vi "Gergberg Setup.vi"() -> ()   [LabVIEW 2012, in "LightPipes.lvlib"]
uses:
  LightPipes.lvlib
panel:
  in  "Target Phase":path=path "C:/Users/Tri/Documents/Lightpipes/LabView/beam images/target_phase.gpl"
  in  "Target PGM":path=path "C:/Users/Tri/Documents/Lightpipes/LabView/beam images/target.pgm"
  in  "R":dbl=0.0001
  in  "size_grid":dbl=0.02
  in  "n_grid":i32=256
  in  "Source Intensity":path=path "C:/Users/Tri/Documents/Lightpipes/LabView/beam images/initial_int.gpl"
  in  "Target Intensity":path=path "C:/Users/Tri/Documents/Lightpipes/LabView/beam images/target_int.gpl"
  in  "PGM gamma":dbl=1.0
  in  "Source PGM":path=path "C:/Users/Tri/Documents/Lightpipes/LabView/beam images/initial.pgm"
  in  "forward distance":dbl=0.5
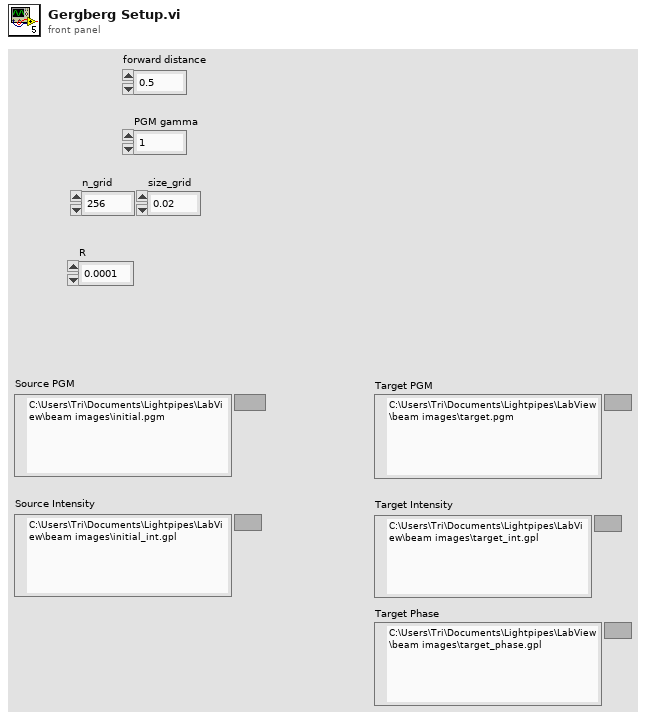
[diagram p1: front panel]
types:
  T1 = cluster{"n_grid":i32, "@dummy control@":i8, "@dummy control@":i8, "@dummy control@":i8, "@dummy control@":i8, "size":dbl, "lambda":dbl, "int1":i32, "int2":i32, "int3":i32, "@dummy control@":i8, "@dummy control@":i8, "@dummy control@":i8, "@dummy control@":i8, "double1":dbl, "double2":dbl, "double3":dbl, "real":u32, "imaginary":u32}
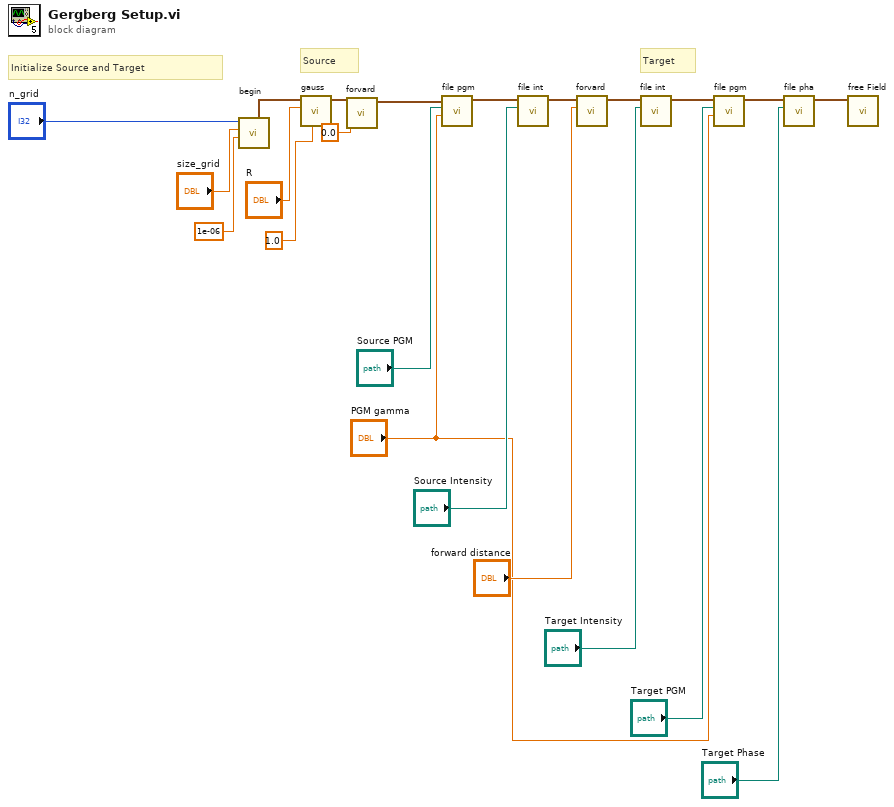
[diagram p0: block diagram]
diagram:
  # "Target"
  # "Source"
  # "Initialize Source and Target"
  n1 = call "begin.vi"("lambda"=1e-06, "size_grid"="size_grid", "n_grid"="n_grid") -> ("field out"=w14:T1)  [unwired: 8 in]
  n2 = call "gauss.vi"("AA"=1.0, "R"="R", "field"=w14) -> ("field out"=w3:T1)  [unwired: 8 in]
  n3 = call "forvard.vi"("distance"=0.0, "field"=w3) -> ("field out"=w2:T1)  [unwired: 9 in]
  n4 = call "file pgm.vi"("gamma"="PGM gamma", "Path"="Source PGM", "field"=w2) -> ("field out"=w13:T1)  [unwired: 7 in, 1 out]
  n5 = call "file int.vi"("Path in"="Source Intensity", "field"=w13) -> ("field out"=w9:T1)  [unwired: 9 in]
  n6 = call "forvard.vi"("distance"="forward distance", "field"=w9) -> ("field out"=w5:T1)  [unwired: 9 in]
  n7 = call "file int.vi"("Path in"="Target Intensity", "field"=w5) -> ("field out"=w18:T1)  [unwired: 9 in]
  n8 = call "file pgm.vi"("gamma"="PGM gamma", "Path"="Target PGM", "field"=w18) -> ("field out"=w17:T1)  [unwired: 7 in, 1 out]
  n9 = call "file pha.vi"("Path in"="Target Phase", "field"=w17) -> ("field out"=w4:T1)  [unwired: 8 in, 1 out]
  n10 = call "free Field.vi"("field"=w4) -> ()  [unwired: 10 in, 1 out]
